vi "Explore to QControl.vi"(8 "error in (no error)":errorcluster, 11 "ControlClassWizard in":refnum<class "QControl Creation Wizard.lvclass">) -> (0 "error out":errorcluster, 3 "ControlClassWizard (dup)":refnum<class "QControl Creation Wizard.lvclass">)   [LabVIEW 2020, in "QControl Creation Wizard.lvclass"]
doc: "<b> </b> <b> </b>\n©2016 Q Software Innovations, LLC (QSI)\nwritten by Quentin Alldredge\nproduced in LabVIEW 2015\n\nsupport@qsoftwareinnovations.com\nwww.qsoftwareinnovations.com\n\nAll rights reserved.\n\nRedistribution and use in source and binary forms, with or without modification, are permitted provided that the following conditions are met:\n\n * Redistributions of source code must retain the above copyright notice, this list of conditions and the following disclaimer.\n * Redistributions in binary form must reproduce the above copyright notice, this list of conditions and the following disclaimer in the documentation and/or other materials provided with the distribution.\n * Neither the name of Q Software Innovations, LLC. nor the names of its contributors may be used to endorse or promote products derived from this software without specific prior written permission.\n\nTHIS SOFTWARE IS PROVIDED BY THE COPYRIGHT HOLDERS AND CONTRIBUTORS \"AS IS\" AND ANY EXPRESS OR IMPLIED WARRANTIES, INCLUDING, BUT NOT LIMITED TO, THE IMPLIED WARRANTIES OF MERCHANTABILITY AND FITNESS FOR A PARTICULAR PURPOSE ARE DISCLAIMED. IN NO EVENT SHALL THE COPYRIGHT OWNER OR CONTRIBUTORS BE LIABLE FOR ANY DIRECT, INDIRECT, INCIDENTAL, SPECIAL, EXEMPLARY, OR CONSEQUENTIAL DAMAGES (INCLUDING, BUT NOT LIMITED TO, PROCUREMENT OF SUBSTITUTE GOODS OR SERVICES; LOSS OF USE, DATA, OR PROFITS; OR BUSINESS INTERRUPTION) HOWEVER CAUSED AND ON ANY THEORY OF LIABILITY, WHETHER IN CONTRACT, STRICT LIABILITY, OR TORT (INCLUDING NEGLIGENCE OR OTHERWISE) ARISING IN ANY WAY OUT OF THE USE OF THIS SOFTWARE, EVEN IF ADVISED OF THE POSSIBILITY OF SUCH DAMAGE."
uses:
  QControl Creation Wizard.lvclass
  QControl Creation Wizard.lvclass/QControl Creation Wizard.ctl
  New QControl Info/New QControl Info.lvclass/New QControl Info.ctl
  New QControl Info/Read New Class Path.vi
  New QControl Info/New QControl Info.lvclass
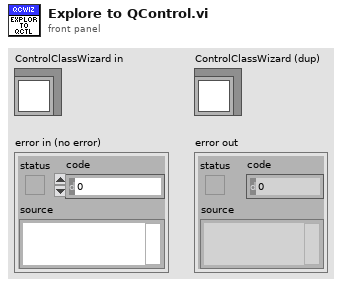
[diagram p1: front panel]
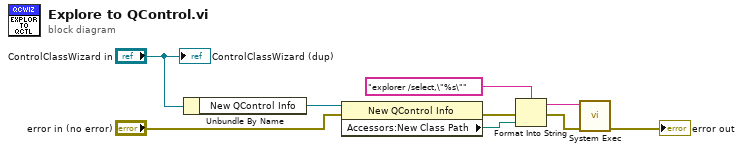
[diagram p0: block diagram]
diagram:
  n1 = Unbundle By Name("ControlClassWizard in") -> ("New QControl Info"=w4:refnum<data-value>)
  n2 = property class="New QControl Info"(reference=w4, error in="error in (no error)") -> (error out=w1:errorcluster, "Accessors:New Class Path"=w3:path)  [unwired: 1 out]
  n3 = Format Into String(format string="explorer /select,\"%s\"", error in=w1, w3) -> (resulting string=w9:string, error out=w6:errorcluster)  [unwired: 1 in]
  n4 = call <vilib>:"System Exec.vi"("error in (no error)"=w6, "command line"=w9) -> ("error out"=→"error out":errorcluster)  [unwired: 6 in, 3 out]
  "ControlClassWizard (dup)" <- "ControlClassWizard in"
